vi "Set Vector.vi"(0 "comm interface in":refnum<class "Pixy Com.lvclass">, 5 "vector":u8, 11 "error in":errorcluster) -> (4 "comm interface out":refnum<class "Pixy Com.lvclass">, 15 "error out":errorcluster)   [LabVIEW 2018, in "Pixy2.lvlib"]
doc: "Selects the index of the vector to use. You must also configure Line Tracking mode to enable vector selection."
uses:
  Pixy2.lvlib
  Interface/Pixy Com.lvclass
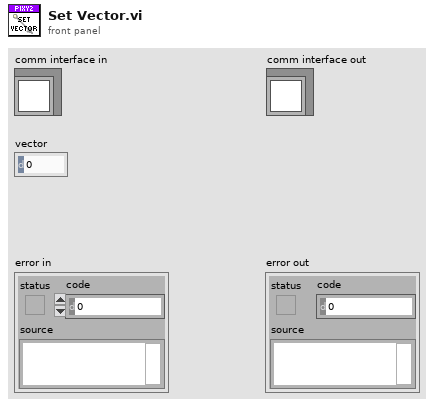
[diagram p1: front panel]
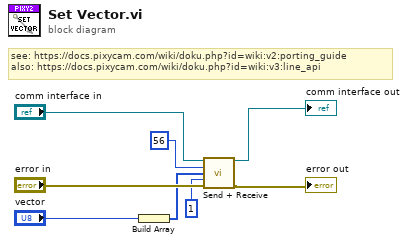
[diagram p0: block diagram]
diagram:
  # "see: https://docs.pixycam.com/wiki/doku.php?id=wiki:v2:porting_guide\nalso: https://docs.pixycam.com/wiki/doku.php?id=wiki:v3:line_api"
  n1 = Build Array("vector") -> (w3:u8[])
  n2 = call "Send + Receive.vi"("comm interface in"="comm interface in", "type"=u8 56, "payload"=w3, "expected response"=u8 1 ("expected type"), "error in"="error in") -> ("comm interface out"=→"comm interface out":refnum<class "Pixy Com.lvclass">, "error out"=→"error out":errorcluster)  [unwired: 8 in, 1 out]
